vi "Aux FIFO demo test.vi"() -> ()   [LabVIEW 2023]
uses:
  <vilib>/eio/EIONode/EIONode.xnode
  <vilib>/rvi/DataTransferAndStorage/Container/XNode/niFpgaContainer.xnode
  <vilib>/rvi/interface/RandomDataEmulation/nirviRandomDataFpgaReadWriteTemplate.vi
  <vilib>/rvi/eio/common/nirviEmuTemplateMethod_errors.vi
panel:
  in  "xt end aux":u32
  in  "stop":bool
  out "elapsed":u32
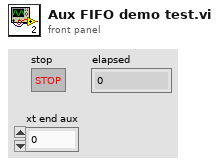
[diagram p1: front panel]
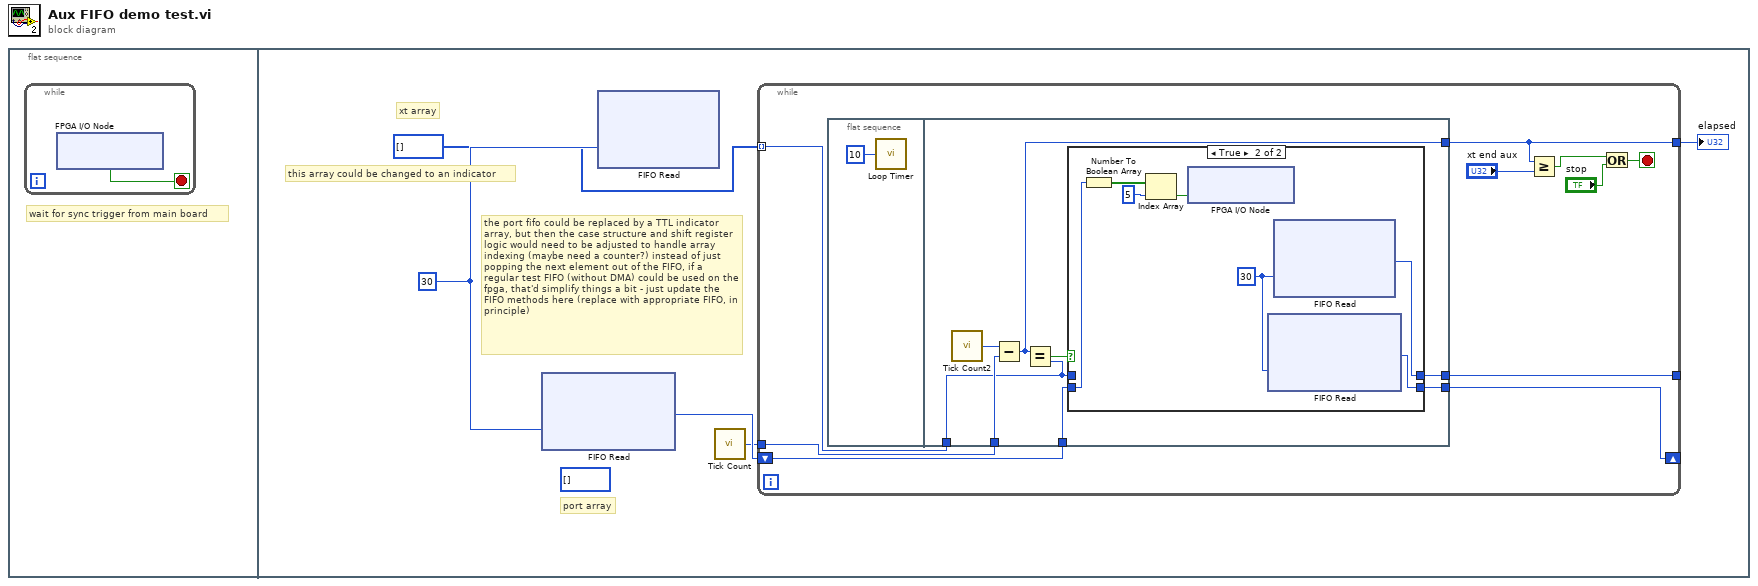
[diagram p0: block diagram]
diagram:
  n1 = flat-sequence {
    frame #0 {
      # "wait for sync trigger from main board"
      n2 = while {
        stop <- w1 stop-if-true
        n3 = xnode "FPGA I/O Node"() -> ("RMC/DIO80"=w1:bool)  [unwired: 1 in, 1 out]
      }
    }
    frame #1 {
      (unwired) i32[] []
      w6 = 30 ("Timeout")
      # "the port fifo could be replaced by a TTL indicator array, but then the case structure and shift register logic would need to be adjusted to handle array indexing (maybe need a counter?) instead of just popping the next element out of the FIFO, if a regular test FIFO (without DMA) could be used on the fpga, that'd simplify things a bit - just update the FIFO methods here (replace with appropriate FIFO, in principle)"
      # "this array could be changed to an indicator"
      # "port array"
      # "xt array"
      n4 = xnode ("FIFO Read")("Timeout"=w6) -> ("Element"=w5:i16)  [unwired: 1 in, 2 out]
      n5 = xnode ("FIFO Read")("Timeout"=w6) -> ()  [unwired: 1 in, 3 out]
      n6 = call "Tick Count"() -> ("Tick Count(uSec)"=w4:u32)
      n7 = while {
        shift-right: [w10] -> _
        shift-left: w5 -> [w12]
        tunnel: w4 -> [w14]
        tunnel: [w7] -> w3
        tunnel: i32[] [] -> [w13] mode=indexing
        tunnel: [w11] -> _
        stop <- w8 stop-if-true
        n8 = flat-sequence {
          tunnel: [w23] -> w7
          tunnel: w14 -> [w22]
          tunnel: w13 -> [w18]
          tunnel: w12 -> [w21]
          tunnel: [w20] -> w11
          tunnel: [w19] -> w10
          frame #0 {
            n9 = call "Loop Timer"("Count(Ticks)"=u32 10 ("Count(mSec)")) -> ()  [unwired: 1 out]
          }
          frame #1 {
            n10 = call "Tick Count2"() -> ("Tick Count(uSec)"=w24:u32)
            n11 = Subtract(x=w24, y=w22) -> (x-y=w23:u32)
            n12 = Equal?(x=w23, y=w18) -> (x = y?=w25:bool)
            n13 = case shown="True" w25 {
              tunnel: [w26 w34] -> w19
              tunnel: [w27 w33] -> w20
              tunnel: w21 -> [w26 w31]
              tunnel: w18 -> [w27 _]
              frame False {
              }
              frame True {
                w30 = i16 30
                n14 = Number To Boolean Array(number=w31) -> (Boolean array=w29:bool[])
                n15 = Index Array(array=w29, index=5) -> (element=w28:bool)
                n16 = xnode "FPGA I/O Node"("RMC/DIO83"=w28) -> ()  [unwired: 1 in, 1 out]
                n17 = xnode ("FIFO Read")("Timeout"=w30) -> ("Element"=w34:i16)  [unwired: 1 in, 2 out]
                n18 = xnode ("FIFO Read")("Timeout"=w30) -> ("Element"=w33:i16)  [unwired: 1 in, 2 out]
              }
            }
          }
        }
        n19 = Greater Or Equal?(x=w7, y="xt end aux") -> (x >= y?=w9:bool)
        n20 = Or(x=w9, y="stop") -> (x .or. y?=w8:bool)
      }
      "elapsed" <- w3
    }
  }
